vi "HMI_ProyectoFinal.vi"() -> ()   [LabVIEW 2018]
uses:
  <vilib>/Platform/TimedLoop/XDataNode/timing_clust.ctl
  <vilib>/Platform/TimedLoop/XDataNode/nitl_modes.ctl
  <vilib>/Platform/TimedLoop/XDataNode/wakeup.ctl
  <vilib>/Instr/_visa.llb/VISA Configure Serial Port (Instr).vi
  <vilib>/Utility/file.llb/Write Delimited Spreadsheet (DBL).vi
  <vilib>/platform/TimedLoop/XDataNode/XDataNode.xnode
  <vilib>/Platform/TimedLoop/XDataNode/XDNodeRunTimeDep.lvlib
panel:
  out "error out":errorcluster
  in  "Tab Control":enum32{"Monitor", "Variables"}(tab)
  out "PLOT5":sgl(graph) caption="Error y Manipulación"
  out "PLOT4":sgl(graph) caption="Error y Manipulación"
  in  "SAVE":bool caption="Guardar Datos"
  in  "STOP":bool
  in  "Log":bool caption="Archivar Datos"
  in  "Ts":dbl=0.05 caption="Muestreo" min=0.1 max=15.0 step=1.0
  in  "Kp":sgl=-15.7 min=0.01
  out "OP":sgl caption="Manipulación" max=100 step=1
  in  "SP":sgl=2.5 caption="Referencia" min=2.5 max=10 step=1
  in  "Ki":sgl=-6.67 min=0.01
  in  "Kd":sgl=-0.06 min=0.01
  out "Error":sgl
  out "PV":sgl
  out "PLOT2":cluster{"OP":sgl, "Error":sgl}(graph) caption="Error y Manipulación"
  out "PLOT1":cluster{"SP":sgl, "PV":sgl}(graph) caption="Variable de Proceso (PV) y Referencia (SP)"
  in  "VISA":refnum<visa-resource-name>
  out "Count":i32 caption="Elementos"
  out "PLOT3":sgl(graph) caption="P"
  in  "Start":bool caption="Iniciar Conexión"
  in  "PWM Period":sgl=7150.0 min=42 max=8000 step=1
  out "D":sgl caption="Kd" min=0.01
  out "I":sgl caption="Ki" min=0.01
  out "P":sgl caption="Kp" min=0.01
  in  "in":string
  in  "timeout":u32=10000
  in  "data bits":u16=8 min=5 max=8 step=1
  in  "parity":enum16{"None", "Odd", "Even", "Mark", "Space"}(ring)
  in  "stop bits":u16(ring)=10 items=["1.0"=10, "1.5"=15, "2.0"=20]
  out "Data":dbl[][](array[numeric])
  in  "flow control":u16(ring) items=["None", "XON/XOFF", "RTS/CTS", "XON/XOFF & RTS/CTS", "DTR/DSR", "XON/XOFF & DTR/DSR"]
  in  "Send Data":bool caption="Guardar Datos"
  out "DataS":u16[](array[numeric])
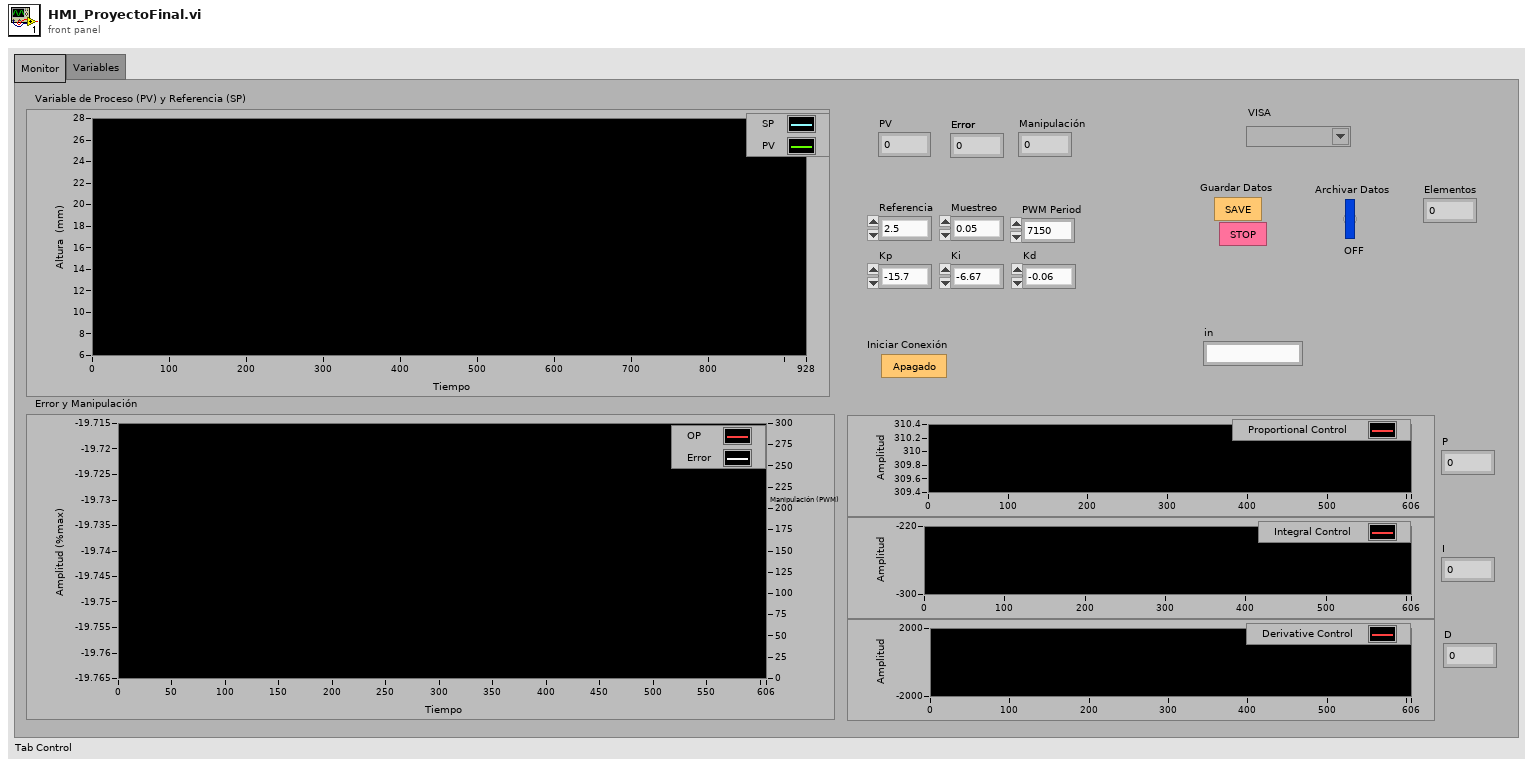
[diagram p1: front panel]
types:
  T1 = typedef "XDNodeRunTimeDep.lvlib/timing_clust.ctl" = cluster{"Expected End [f-1]":u64, "Actual End [f-1]":u64, "Finished Late? [f-1]":bool, "Expected End [i-1]":u64, "Actual End [i-1]":u64, "Finished Late? [i-1]":bool, "Expected Start [i]":u64, "Actual Start [i]":u64, "Expected Start [f]":u64, "Actual Start [f]":u64, "Source Name":string, "Structure Name":string, "Period":i64, "Deadline":i64, "Offset":i64, "Start":i64, "Priority":i32, "Timeout":i32, "Mode":T2, "Wakeup Reason":T3, "Error":errorcluster, "Source Type":string, "Secondary Source Type":string, "Global End Time":u64, "Global Start Time":u64, "Frame Duration":u64, "Iteration Duration":u64, "Assigned CPU":i32, "I/O Scan Engine Mode":u32}
  T2 = typedef "XDNodeRunTimeDep.lvlib/nitl_modes.ctl" = enum32{"No Change", "Process missed periods, maintain original phase", "Discard missed periods, maintain original phase", "Process missed periods, ignore original phase", "Discard missed periods, ignore original phase"}
  T3 = typedef "XDNodeRunTimeDep.lvlib/wakeup.ctl" = enum32{"Normal", "Aborted", "Asynchronous wakeup", "Timing source error", "Timed loop error", "Timeout"}
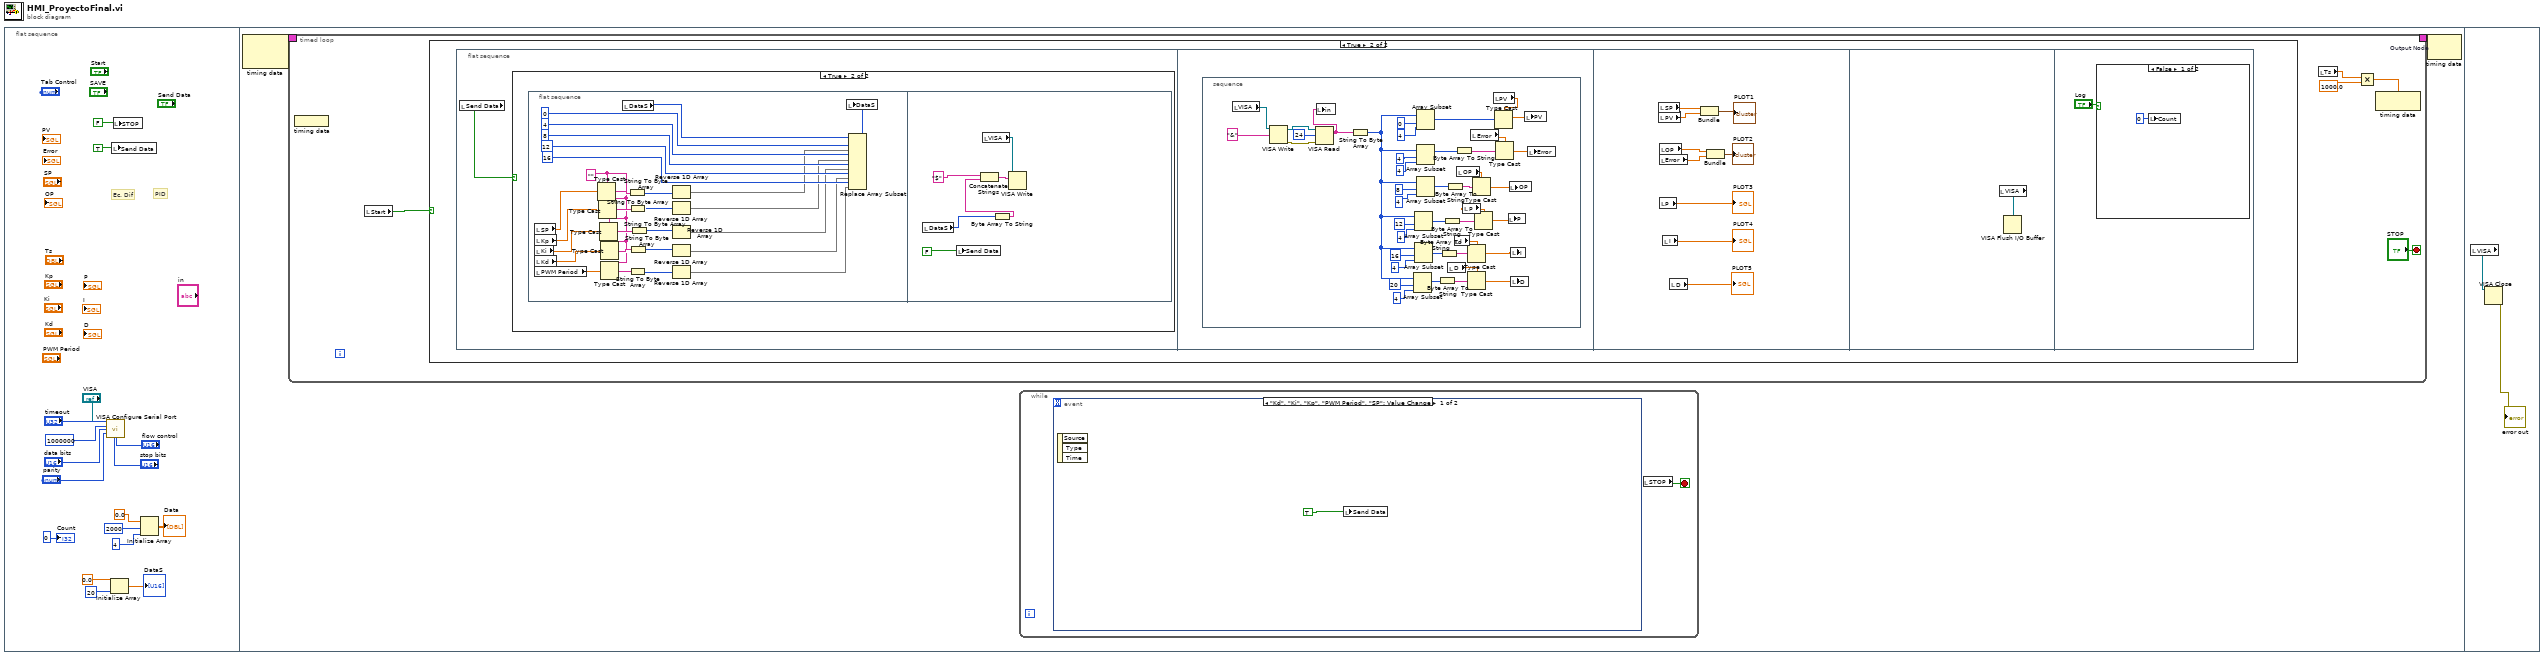
[diagram p0: block diagram]
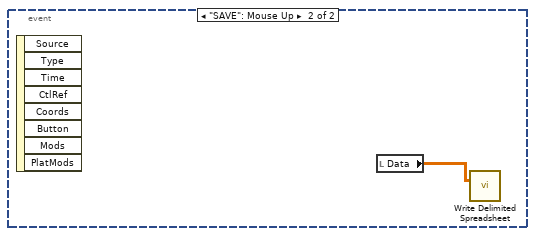
[diagram p2: hidden frame]
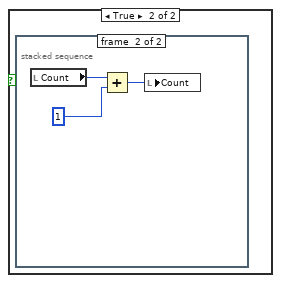
[diagram p5: hidden frame]
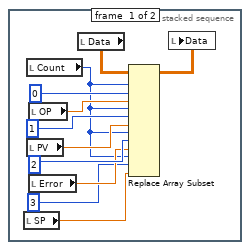
[diagram p6: hidden frame]
diagram:
  n1 = flat-sequence {
    frame #0 {
      # "Ec. Dif"
      # "PID"
      n2 = call-poly "VISA Configure Serial Port"("VISA resource name"="VISA", "timeout (10sec)"="timeout", "baud rate (9600)"=u64 1000000 ("baud rate"), "data bits (8)"="data bits", "parity (0:none)"="parity", "stop bits (10: 1 bit)"="stop bits", "flow control (0:none)"="flow control") -> ()  [unwired: 7 in, 2 out]
      n3 = Initialize Array(0.0, 20) -> (→"DataS":dbl[])
      n4 = local write "Send Data"(TRUE) -> ()
      n5 = local write "STOP"(FALSE) -> ()
      n6 = Initialize Array(0.0, 2000, 4) -> (→"Data":dbl[][])
      "Count" <- 0
    }
    frame #1 {
      n7 = node-c288() -> (w19:T1)  [unwired: 2 in]
      n8 = timed-loop {
        timing: w19 -> [_]
        timing-out: [_] -> w18
        stop <- "STOP" stop-if-true
        n9 = node-c288() -> ()  [unwired: 1 in]
        n10 = local read "Start"() -> (w23:bool)
        n11 = case shown="True" w23 {
          frame False {
          }
          frame True {
            n12 = flat-sequence {
              frame #0 {
                n13 = local read "Send Data"() -> (w28:bool)
                n14 = case shown="True" w28 {
                  frame False {
                  }
                  frame True {
                    n15 = flat-sequence {
                      frame #0 {
                        w39 = "" ("type")
                        n16 = local read "SP"() -> (w49:sgl)
                        n17 = local read "Kp"() -> (w47:sgl)
                        n18 = local read "Ki"() -> (w45:sgl)
                        n19 = local read "Kd"() -> (w41:sgl)
                        n20 = local read "PWM Period"() -> (w42:sgl)
                        n21 = Type Cast(type=w39, x=w49) -> (*(type *) &x=w48:string)
                        n22 = Type Cast(type=w39, x=w47) -> (*(type *) &x=w46:string)
                        n23 = Type Cast(type=w39, x=w45) -> (*(type *) &x=w44:string)
                        n24 = Type Cast(type=w39, x=w42) -> (*(type *) &x=w40:string)
                        n25 = Type Cast(type=w39, x=w41) -> (*(type *) &x=w43:string)
                        n26 = local read "DataS"() -> (w55:u16[])
                        n27 = String To Byte Array(string=w48) -> (unsigned byte array=w36:u8[])
                        n28 = String To Byte Array(string=w46) -> (unsigned byte array=w35:u8[])
                        n29 = String To Byte Array(string=w40) -> (unsigned byte array=w38:u8[])
                        n30 = String To Byte Array(string=w43) -> (unsigned byte array=w33:u8[])
                        n31 = String To Byte Array(string=w44) -> (unsigned byte array=w34:u8[])
                        n32 = Reverse 1D Array(array=w35) -> (reversed array=w30:u8[])
                        n33 = Reverse 1D Array(array=w34) -> (reversed array=w31:u8[])
                        n34 = Reverse 1D Array(array=w33) -> (reversed array=w32:u8[])
                        n35 = Reverse 1D Array(array=w38) -> (reversed array=w37:u8[])
                        n36 = Reverse 1D Array(array=w36) -> (reversed array=w29:u8[])
                        n37 = Replace Array Subset(array=w55, new element #1=w29, index #1=0, new element #2=w30, index #2=4, new element #3=w31, index #3=8, new element #4=w32, index #4=12, new element #5=w37, index #5=16) -> (w56:u16[])
                        n38 = local write "DataS"(w56) -> ()
                      }
                      frame #1 {
                        n39 = local read "DataS"() -> (w58:u16[])
                        n40 = local write "Send Data"(FALSE) -> ()
                        n41 = local read "VISA"() -> (w62:refnum<visa-resource-name>)
                        n42 = Byte Array To String(unsigned byte array=w58) -> (string=w57:string)
                        n43 = Concatenate Strings("$" ("type"), w57) -> (w60:string)
                        n44 = VISA Write(VISA resource name=w62, write buffer=w60) -> ()  [unwired: 1 in, 3 out]
                      }
                    }
                  }
                }
              }
              frame #1 {
                n45 = stacked-sequence {
                  frame #0 {
                    n46 = local read "VISA"() -> (w104:refnum<visa-resource-name>)
                    n47 = VISA Write(VISA resource name=w104, write buffer="&" ("type")) -> (VISA resource name out=w103:refnum<visa-resource-name>, error out=w102:errorcluster)  [unwired: 1 in, 1 out]
                    n48 = VISA Read(VISA resource name=w103, byte count=24, error in (no error)=w102) -> (read buffer=w78:string)  [unwired: 3 out]
                    n49 = local write "in"(w78) -> ()
                    n50 = String To Byte Array(string=w78) -> (unsigned byte array=w99:u8[])
                    n51 = Array Subset(array=w99, index=20, length=4) -> (w76:u8[])
                    n52 = Array Subset(array=w99, index=12, length=4) -> (w73:u8[])
                    n53 = Array Subset(array=w99, index=16, length=4) -> (w75:u8[])
                    n54 = Array Subset(array=w99, index=8, length=4) -> (w71:u8[])
                    n55 = Array Subset(array=w99, index=0, length=4) -> (w63:u8[])
                    n56 = Array Subset(array=w99, index=4, length=4) -> (w69:u8[])
                    n57 = Byte Array To String(unsigned byte array=w76) -> (string=w77:string)
                    n58 = Byte Array To String(unsigned byte array=w75) -> (string=w74:string)
                    n59 = Byte Array To String(unsigned byte array=w73) -> (string=w72:string)
                    n60 = Byte Array To String(unsigned byte array=w71) -> (string=w70:string)
                    n61 = local read "D"() -> (w64:sgl)
                    n62 = local read "I"() -> (w65:sgl)
                    n63 = Byte Array To String(unsigned byte array=w69) -> (string=w68:string)
                    n64 = local read "OP"() -> (w67:sgl)
                    n65 = local read "P"() -> (w66:sgl)
                    n66 = Type Cast(type=w65, x=w74) -> (*(type *) &x=w83:sgl)
                    n67 = Type Cast(type=w64, x=w77) -> (*(type *) &x=w82:sgl)
                    n68 = local read "Error"() -> (w79:sgl)
                    n69 = Type Cast(type=w67, x=w70) -> (*(type *) &x=w85:sgl)
                    n70 = Type Cast(type=w66, x=w72) -> (*(type *) &x=w84:sgl)
                    n71 = local read "PV"() -> (w80:sgl)
                    n72 = Type Cast(type=w80, x=w63) -> (*(type *) &x=w81:sgl)
                    n73 = Type Cast(type=w79, x=w68) -> (*(type *) &x=w86:sgl)
                    n74 = local write "P"(w84) -> ()
                    n75 = local write "OP"(w85) -> ()
                    n76 = local write "I"(w83) -> ()
                    n77 = local write "D"(w82) -> ()
                    n78 = local write "PV"(w81) -> ()
                    n79 = local write "Error"(w86) -> ()
                  }
                }
              }
              frame #2 {
                n80 = local read "SP"() -> (w110:sgl)
                n81 = local read "PV"() -> (w108:sgl)
                n82 = local read "OP"() -> (w111:sgl)
                n83 = local read "Error"() -> (w112:sgl)
                n84 = local read "P"() -> (→"PLOT3":sgl)
                n85 = local read "I"() -> (→"PLOT4":sgl)
                n86 = local read "D"() -> (→"PLOT5":sgl)
                n87 = Bundle("SP"=w110, "PV"=w108) -> (→"PLOT1":cluster{"SP":sgl, "PV":sgl})  [unwired: 1 in]
                n88 = Bundle("OP"=w111, "Error"=w112) -> (→"PLOT2":cluster{"OP":sgl, "Error":sgl})  [unwired: 1 in]
              }
              frame #3 {
                n89 = local read "VISA"() -> (w114:refnum<visa-resource-name>)
                n90 = VISA Flush I/O Buffer(VISA resource name=w114) -> ()  [unwired: 2 in, 2 out]
              }
              frame #4 {
                n91 = case shown="False" "Log" {
                  frame False {
                    n92 = local write "Count"(0 ("Count")) -> ()
                  }
                  frame True {
                    n93 = stacked-sequence {
                      frame #0 {
                        n94 = local read "SP"() -> (w118:sgl)
                        n95 = local read "Count"() -> (w119:i32)
                        n96 = local read "PV"() -> (w123:sgl)
                        n97 = local read "OP"() -> (w124:sgl)
                        n98 = local read "Error"() -> (w120:sgl)
                        n99 = local read "Data"() -> (w127:dbl[][])
                        n100 = Replace Array Subset(array=w127, new element #1=w124, index (row) #1=w119, index (col) #1=0, new element #2=w123, index (row) #2=w119, index (col) #2=1 ("disabled index (col)"), new element #3=w120, index (row) #3=w119, index (col) #3=2, new element #4=w118, index (row) #4=w119, index (col) #4=3) -> (w126:dbl[][])
                        n101 = local write "Data"(w126) -> ()
                      }
                      frame #1 {
                        n102 = local read "Count"() -> (w130:i32)
                        n103 = Add(x=w130, y=1) -> (x+y=w128:i32)
                        n104 = local write "Count"(w128) -> ()
                      }
                    }
                  }
                }
              }
            }
          }
        }
        n105 = local read "Ts"() -> (w25:dbl)
        n106 = Multiply(x=w25, y=1000.0) -> (x*y=w26:dbl)
        n107 = node-c288(w26) -> ()  [unwired: 1 out]
      }
      n108 = while {
        stop <- w20 stop-if-true
        n109 = event shown="[0] \"Kd\", \"Ki\", \"Kp\", \"PWM Period\", \"SP\": Value Change" {
          selector: _ -> [_ _]
          dyn-events: _ -> [_ _]
          timeout: _ -> [_ _]
          event "Kd", "Ki", "Kp", "PWM Period", "SP": Value Change {
            n110 = event-data() -> ()  [unwired: 1 in, 3 out]
            n111 = local write "Send Data"(TRUE) -> ()
          }
          event "SAVE": Mouse Up {
            n112 = event-data() -> ()  [unwired: 1 in, 8 out]
            n113 = local read "Data"() -> (w22:dbl[][])
            n114 = call-poly <vilib>:"Write Delimited Spreadsheet.vi"("2D data"=w22) -> ()  [unwired: 13 in, 2 out]
          }
        }
        n115 = local read "STOP"() -> (w20:bool)
      }
      n116 = node-c288 "Output Node"(w18) -> ()  [unwired: 1 out]
    }
    frame #2 {
      n117 = local read "VISA"() -> (w138:refnum<visa-resource-name>)
      n118 = VISA Close(VISA resource name=w138) -> (error out=→"error out":errorcluster)  [unwired: 1 in]
    }
  }
